vi "Destroy Buffer.vi"(8 "error in":errorcluster, 9 "Return Elements (T)":bool=TRUE, 11 "Buffer":refnum<data-value>) -> (0 "error out":errorcluster, 2 "elements":variant[](array[variant]))   [LabVIEW 2013, in "VariantBuffer.lvclass"]
doc: "This VI releases resources that have been created for the ring buffer."
uses:
  VariantBuffer.lvclass
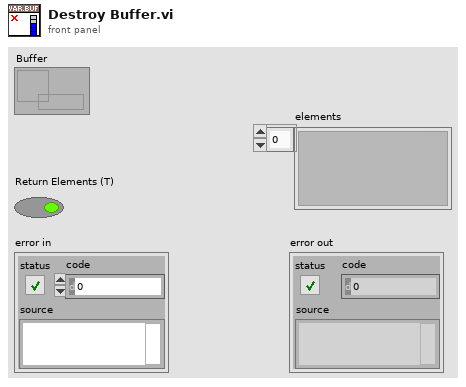
[diagram p1: front panel]
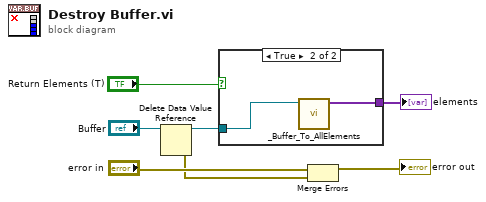
[diagram p0: block diagram]
diagram:
  n1 = Delete Data Value Reference(data value reference="Buffer") -> (data value=w6:refnum<class "VariantBuffer.lvclass">, error out=w2:errorcluster)  [unwired: 1 in]
  n2 = case shown="True" "Return Elements (T)" {
    tunnel: w6 -> [_ w9]
    tunnel: [_ w8] -> w5
    frame False {
    }
    frame True {
      n3 = call "_Buffer_To_AllElements.vi"("Buffer"=w9) -> ("elements"=w8:variant[])  [unwired: 10 in]
    }
  }
  "elements" <- w5
  n4 = Merge Errors("error in", w2) -> (→"error out":errorcluster)
